vi "TCP-Send Command (CRLF).vi"(0 "PXI Address":string, 5 "Port":i32, 7 "Command":string, 9 "timeout (ms)":i32=5000, 11 "error in (no error)":errorcluster, 12 "fast response":bool) -> (15 "error out":errorcluster)   [LabVIEW 2015]
panel:
  out "result":i32
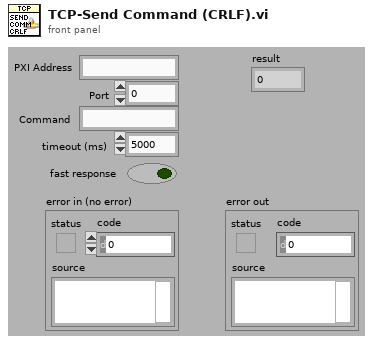
[diagram p1: front panel]
types:
  T1 = enum16{"Standard", "Buffered", "CRLF", "Immediate"}
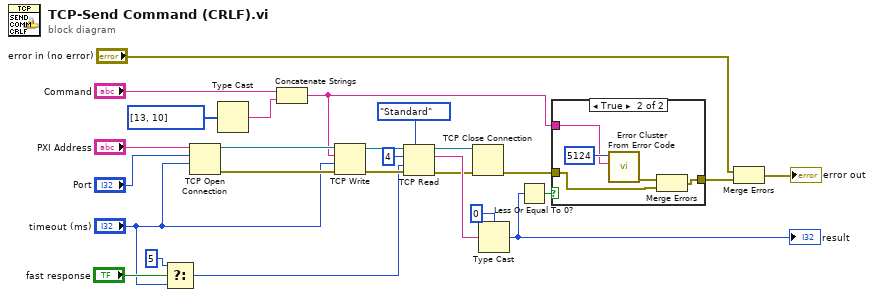
[diagram p0: block diagram]
diagram:
  n1 = Select(t=5 ("timeout ms (25000)"), s="fast response", f="timeout (ms)") -> (s? t:f=w6:i32)
  n2 = TCP Open Connection(address="PXI Address", remote port or service name="Port", timeout ms (60000)="timeout (ms)") -> (connection ID=w24:refnum<k5>, error out=w13:errorcluster)  [unwired: 2 in]
  n3 = Type Cast(x=u8[] [13, 10]) -> (*(type *) &x=w1:string)  [unwired: 1 in]
  n4 = Concatenate Strings("Command", w1) -> (w2:string)
  n5 = TCP Write(connection ID=w24, data in=w2, error in (no error)=w13, 9:"timeout (ms)") -> (connection ID out=w23:refnum<k5>, error out=w10:errorcluster)  [unwired: 1 out]
  n6 = TCP Read(connection ID=w23, bytes to read=4, error in (no error)=w10, 7:T1."Standard" ("mode (standard)"), 9:w6) -> (connection ID out=w22:refnum<k5>, data out=w21:string, error out=w9:errorcluster)
  n7 = TCP Close Connection(connection ID=w22, error in (no error)=w9) -> (error out=w12:errorcluster)  [unwired: 1 in, 1 out]
  n8 = Type Cast(type=0, x=w21) -> (*(type *) &x=w4:i32)
  "result" <- w4
  n9 = Less Or Equal To 0?(x=w4) -> (x <= 0?=w19:bool)
  n10 = case shown="True" w19 {
    tunnel: [w27 w29] -> w17
    tunnel: w12 -> [w27 w28]
    tunnel: w2 -> [_ w30]
    frame False {
    }
    frame True {
      n11 = call <vilib>:"Error Cluster From Error Code.vi"("error message (\"\")"=w30, "error code (0)"=5124) -> ("error out"=w32:errorcluster)  [unwired: 7 in]
      n12 = Merge Errors(w32, w28) -> (w29:errorcluster)
    }
  }
  n13 = Merge Errors("error in (no error)", w17) -> (→"error out":errorcluster)
